vi "Read StartServer.vi"(8 "error in (no error)":errorcluster caption="错误输入（无错误）", 11 "MQTT_Server_Actor输入":refnum<class "MQTT_Server_Actor.lvclass">) -> (0 "error out":errorcluster caption="错误输出", 2 "StartServer":refnum<user-event>, 3 "MQTT_Server_Actor输出":refnum<class "MQTT_Server_Actor.lvclass">)   [LabVIEW 2018, in "MQTT_Server_Actor.lvlib" / "MQTT_Server_Actor.lvclass"]
uses:
  MQTT_Server_Actor.lvclass
  StartServer.ctl
  MQTT_Server_Actor.lvclass/MQTT_Server_Actor.ctl
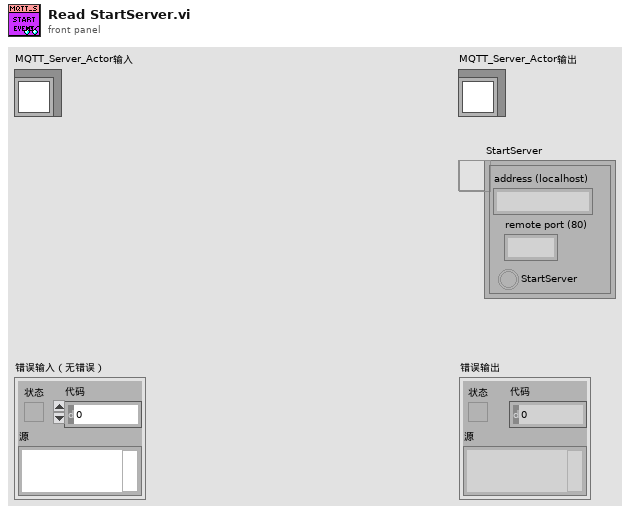
[diagram p1: front panel]
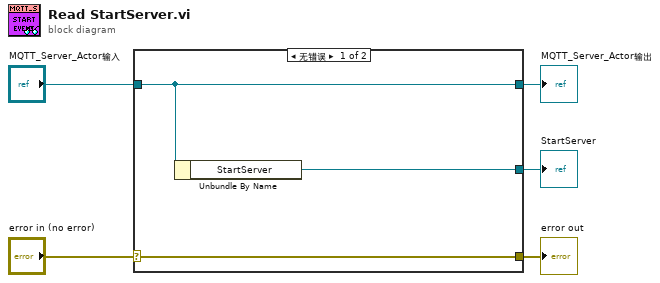
[diagram p0: block diagram]
diagram:
  n1 = case shown="无错误" "error in (no error)" {
    selector: "error in (no error)" -> [w8 w9]
    tunnel: [w8 w9] -> w4
    tunnel: [w7 w10] -> w2
    tunnel: "MQTT_Server_Actor输入" -> [w7 w10]
    tunnel: [w6 _] -> w1
    frame No Error {
      n2 = Unbundle By Name(w7) -> ("StartServer"=w6:refnum<user-event>)
    }
    frame Error {
    }
  }
  "error out" <- w4
  "MQTT_Server_Actor输出" <- w2
  "StartServer" <- w1
